vi "QAQC.vi"() -> ()   [LabVIEW 2015]
uses:
  global_qaqc.vi
  Global_mitu.vi
panel:
  in  "New Session":bool
  in  "Stop Button":bool
  in  "Tab Control":T1(tab)
  in  "Piralux DX test (Picoammeter)":bool
  out "Check fatti?":bool
  in  "Incollaggio Boccole e Interconnessioni":bool
  in  "Riparazione Pillars":bool
  in  "Piralux SX test (Picoammeter)":bool
  in  "Resistive strips test (Keithley)":bool
  in  "Lavaggio":bool
  in  "Ispezione visiva":bool
  in  "Check Data Sheet":bool
  in  "Name of the PCB":string
  in  "Linear height":bool
  in  "Pass/Not pass":bool
  in  "Pass/Not pass Cooling Bars":bool
  in  "Name of theFoil":string
  in  "Take Measures (Mitutoyo)":bool
  # "Guide to frame QAQC:\n\n1) Visual Inspection\n\n\n\n\n\n\n2) Pass/Not pass check\n\n\n\n\n\n3) Linear height measurement\n\n\n\n\n\n4) Washing\n\n\n\n\n\n5) Storage"
  # "a) Visually check the frames on all sides to verify dents or metallic shavings\nb) Check if the ends of the frames on all sides are planar and file them if not\nc) If the ends were filed, use the air compressore to get rid of the dust on the frames\nd) Check frame planarity by positioning and pressing it against the table"
  # "Throroughly wash the frames with water and saop and let them dry"
  # "Store the frames in the dedicated box"
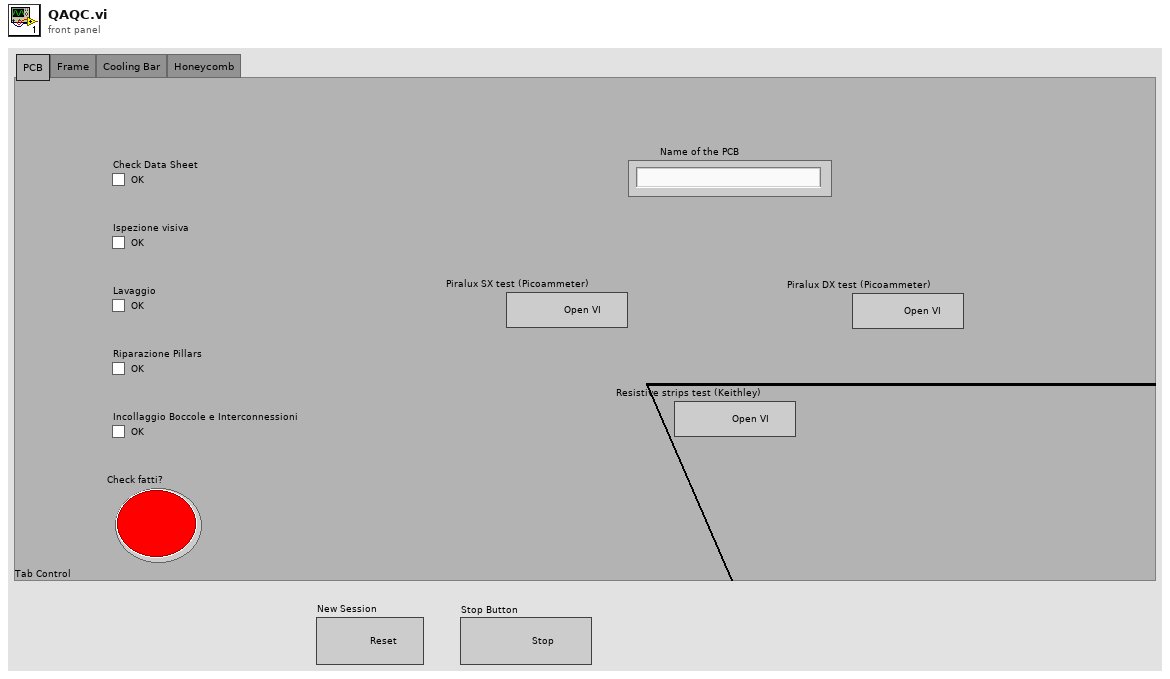
[diagram p1: front panel]
types:
  T1 = enum32{"PCB", "Frame", "Cooling Bar", "Honeycomb"}
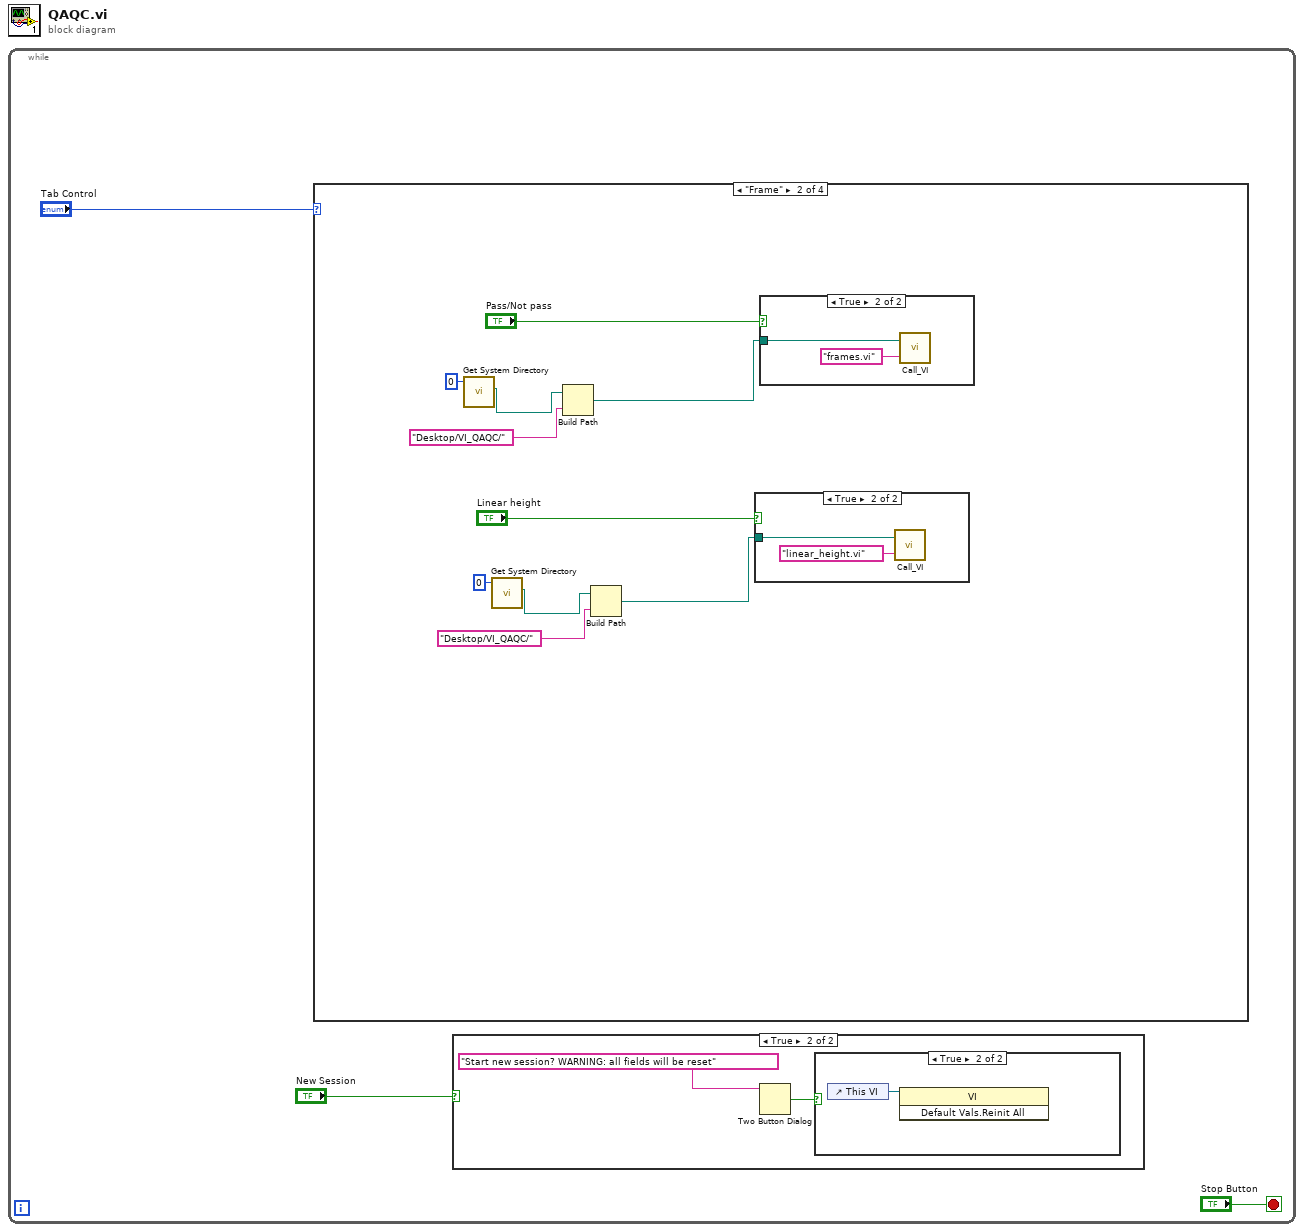
[diagram p0: block diagram]
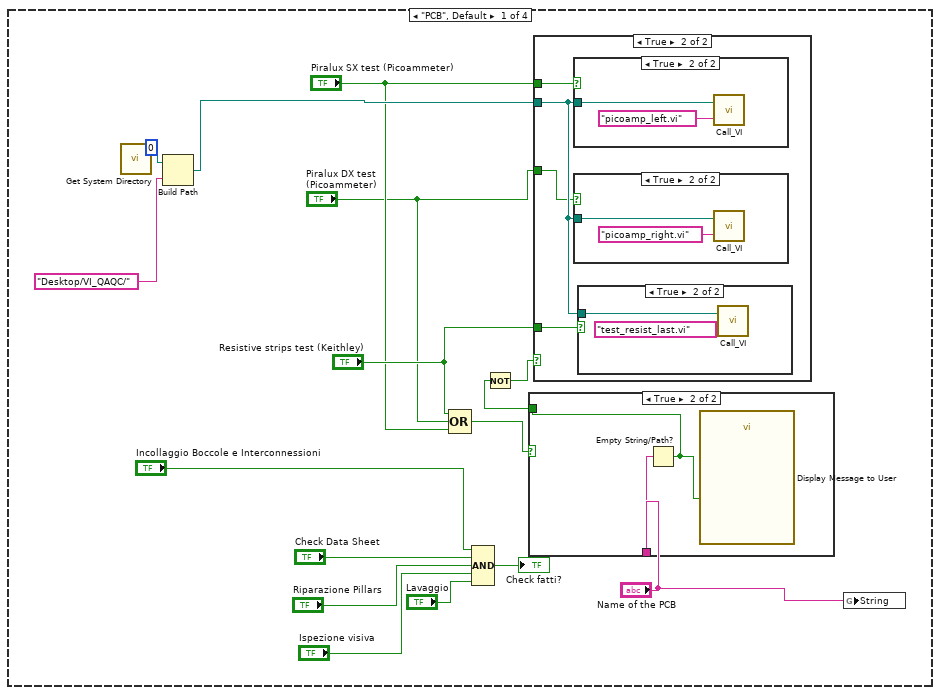
[diagram p4: hidden frame]
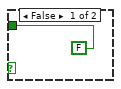
[diagram p9: hidden frame]
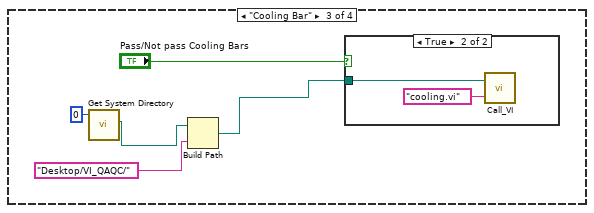
[diagram p12: hidden frame]
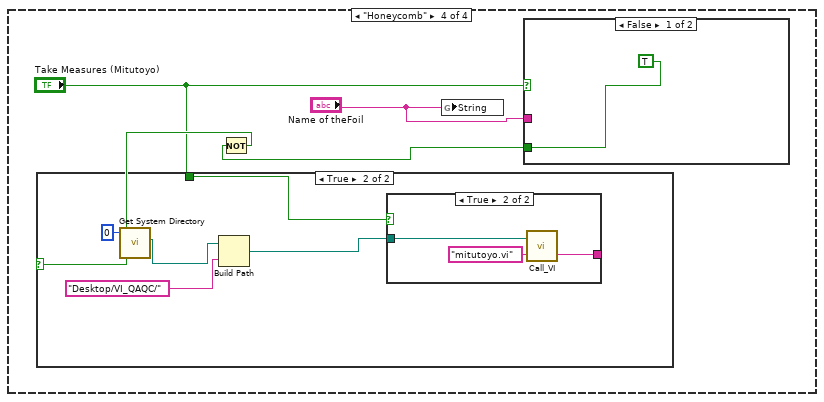
[diagram p14: hidden frame]
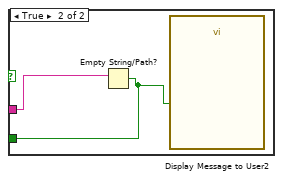
[diagram p15: hidden frame]
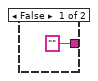
[diagram p17: hidden frame]
diagram:
  n1 = while {
    stop <- "Stop Button" stop-if-true
    n2 = case shown="\"Frame\"" "Tab Control" {
      frame "PCB", Default {
        n3 = call <vilib>:"Get System Directory.vi"("system directory type"=0) -> ("system directory"=w16:path)  [unwired: 10 in]
        n4 = Build Path(base path=w16, name or relative path="Desktop/VI_QAQC/") -> (appended path=w15:path)
        n5 = Compound Arithmetic op=OR("Resistive strips test (Keithley)", "Piralux DX test (Picoammeter)", "Piralux SX test (Picoammeter)") -> (w12:bool)
        n6 = Compound Arithmetic op=AND("Incollaggio Boccole e Interconnessioni", "Check Data Sheet", "Riparazione Pillars", "Ispezione visiva", "Lavaggio") -> (→"Check fatti?":bool)
        n7 = case shown="True" w12 {
          tunnel: "Name of the PCB" -> [_ w36]
          tunnel: [FALSE w35] -> w8
          frame False {
          }
          frame True {
            n8 = Empty String/Path?(string/path=w36) -> (empty?=w35:bool)
            n9 = call "Display Message to User"("Enable"=w35) -> ()  [unwired: 9 in, 2 out]
          }
        }
        n10 = Not(x=w8) -> (.not. x?=w9:bool)
        n11 = case shown="True" w9 {
          tunnel: w15 -> [_ w27]
          tunnel: "Resistive strips test (Keithley)" -> [_ w26]
          tunnel: "Piralux SX test (Picoammeter)" -> [_ w25]
          tunnel: "Piralux DX test (Picoammeter)" -> [_ w24]
          frame False {
          }
          frame True {
            n12 = case shown="True" w25 {
              tunnel: w27 -> [_ w30]
              frame False {
              }
              frame True {
                n13 = call "Call_VI.vi"("Target VI"="picoamp_left.vi", "File Path Control"=w30) -> ()  [unwired: 2 out]
              }
            }
            n14 = case shown="True" w24 {
              tunnel: w27 -> [_ w28]
              frame False {
              }
              frame True {
                n15 = call "Call_VI.vi"("Target VI"="picoamp_right.vi", "File Path Control"=w28) -> ()  [unwired: 2 out]
              }
            }
            n16 = case shown="True" w26 {
              tunnel: w27 -> [_ w32]
              frame False {
              }
              frame True {
                n17 = call "Call_VI.vi"("Target VI"="test_resist_last.vi", "File Path Control"=w32) -> ()  [unwired: 2 out]
              }
            }
          }
        }
        n18 = global write "global_qaqc.vi" "String"("Name of the PCB") -> ()
      }
      frame "Frame" {
        n19 = call <vilib>:"Get System Directory.vi"("system directory type"=0) -> ("system directory"=w43:path)  [unwired: 10 in]
        n20 = call <vilib>:"Get System Directory.vi"("system directory type"=0) -> ("system directory"=w40:path)  [unwired: 10 in]
        n21 = Build Path(base path=w43, name or relative path="Desktop/VI_QAQC/") -> (appended path=w38:path)
        n22 = Build Path(base path=w40, name or relative path="Desktop/VI_QAQC/") -> (appended path=w37:path)
        n23 = case shown="True" "Linear height" {
          tunnel: w37 -> [_ w47]
          frame False {
          }
          frame True {
            n24 = call "Call_VI.vi"("Target VI"="linear_height.vi", "File Path Control"=w47) -> ()  [unwired: 2 out]
          }
        }
        n25 = case shown="True" "Pass/Not pass" {
          tunnel: w38 -> [_ w49]
          frame False {
          }
          frame True {
            n26 = call "Call_VI.vi"("Target VI"="frames.vi", "File Path Control"=w49) -> ()  [unwired: 2 out]
          }
        }
      }
      frame "Cooling Bar" {
        n27 = call <vilib>:"Get System Directory.vi"("system directory type"=0) -> ("system directory"=w53:path)  [unwired: 10 in]
        n28 = Build Path(base path=w53, name or relative path="Desktop/VI_QAQC/") -> (appended path=w51:path)
        n29 = case shown="True" "Pass/Not pass Cooling Bars" {
          tunnel: w51 -> [_ w56]
          frame False {
          }
          frame True {
            n30 = call "Call_VI.vi"("Target VI"="cooling.vi", "File Path Control"=w56) -> ()  [unwired: 2 out]
          }
        }
      }
      frame "Honeycomb" {
        n31 = global write "Global_mitu.vi" "String"("Name of theFoil") -> ()
        n32 = case shown="False" "Take Measures (Mitutoyo)" {
          tunnel: [TRUE w63] -> w60
          tunnel: "Name of theFoil" -> [_ w64]
          frame False {
          }
          frame True {
            n33 = Empty String/Path?(string/path=w64) -> (empty?=w63:bool)
            n34 = call "Display Message to User2"("Enable"=w63) -> ()  [unwired: 9 in, 2 out]
          }
        }
        n35 = Not(x=w60) -> (.not. x?=w61:bool)
        n36 = case shown="True" w61 {
          tunnel: "Take Measures (Mitutoyo)" -> [_ w69]
          frame False {
          }
          frame True {
            n37 = call <vilib>:"Get System Directory.vi"("system directory type"=0) -> ("system directory"=w67:path)  [unwired: 10 in]
            n38 = Build Path(base path=w67, name or relative path="Desktop/VI_QAQC/") -> (appended path=w65:path)
            n39 = case shown="True" w69 {
              tunnel: ["" ("String") w72] -> _
              tunnel: w65 -> [_ w71]
              frame False {
              }
              frame True {
                n40 = call "Call_VI.vi"("Target VI"="mitutoyo.vi", "File Path Control"=w71) -> ("String"=w72:string)  [unwired: 1 out]
              }
            }
          }
        }
      }
    }
    n41 = case shown="True" "New Session" {
      frame False {
      }
      frame True {
        n42 = Two Button Dialog(message="Start new session? WARNING: all fields will be reset") -> (T button?=w4:bool)  [unwired: 2 in]
        n43 = case shown="True" w4 {
          frame False {
          }
          frame True {
            n44 = control-ref of="This VI"() -> (w6:refnum<vi>)
            n45 = invoke class="VI" method="Default Vals.Reinit All"(reference=w6) -> ()  [unwired: 2 in, 3 out]
          }
        }
      }
    }
  }
